vi "API.vi"(8 "error in (no error)":errorcluster, 11 "DataHandlerTask in":refnum<class "DataHandlerTask.lvclass">) -> (0 "error out":errorcluster, 2 "API":refnum<class "API.lvclass">, 3 "DataHandlerTask out":refnum<class "DataHandlerTask.lvclass">)   [LabVIEW 2020, in "Volatus.lvlib" / "DataHandlerTask.lvclass"]
uses:
  DataHandlerTask.lvclass
  API/API.lvclass
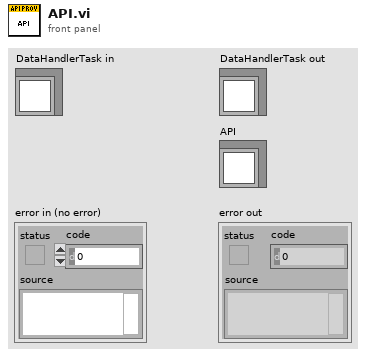
[diagram p1: front panel]
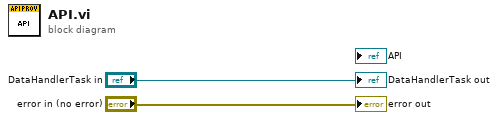
[diagram p0: block diagram]
diagram:
  "error out" <- "error in (no error)"
  "DataHandlerTask out" <- "DataHandlerTask in"
